vi "Extract Previous Sensor Locations.vi"(8 "error in (no error)":errorcluster, 11 "Folder Path":path) -> (0 "error out":errorcluster, 2 "Smoothness Exam Text":string[][](array[string]), 3 "Sensors":string[][](array[string]))   [LabVIEW 2020]
uses:
  <vilib>/regexp/Match Regular Expression.xnode
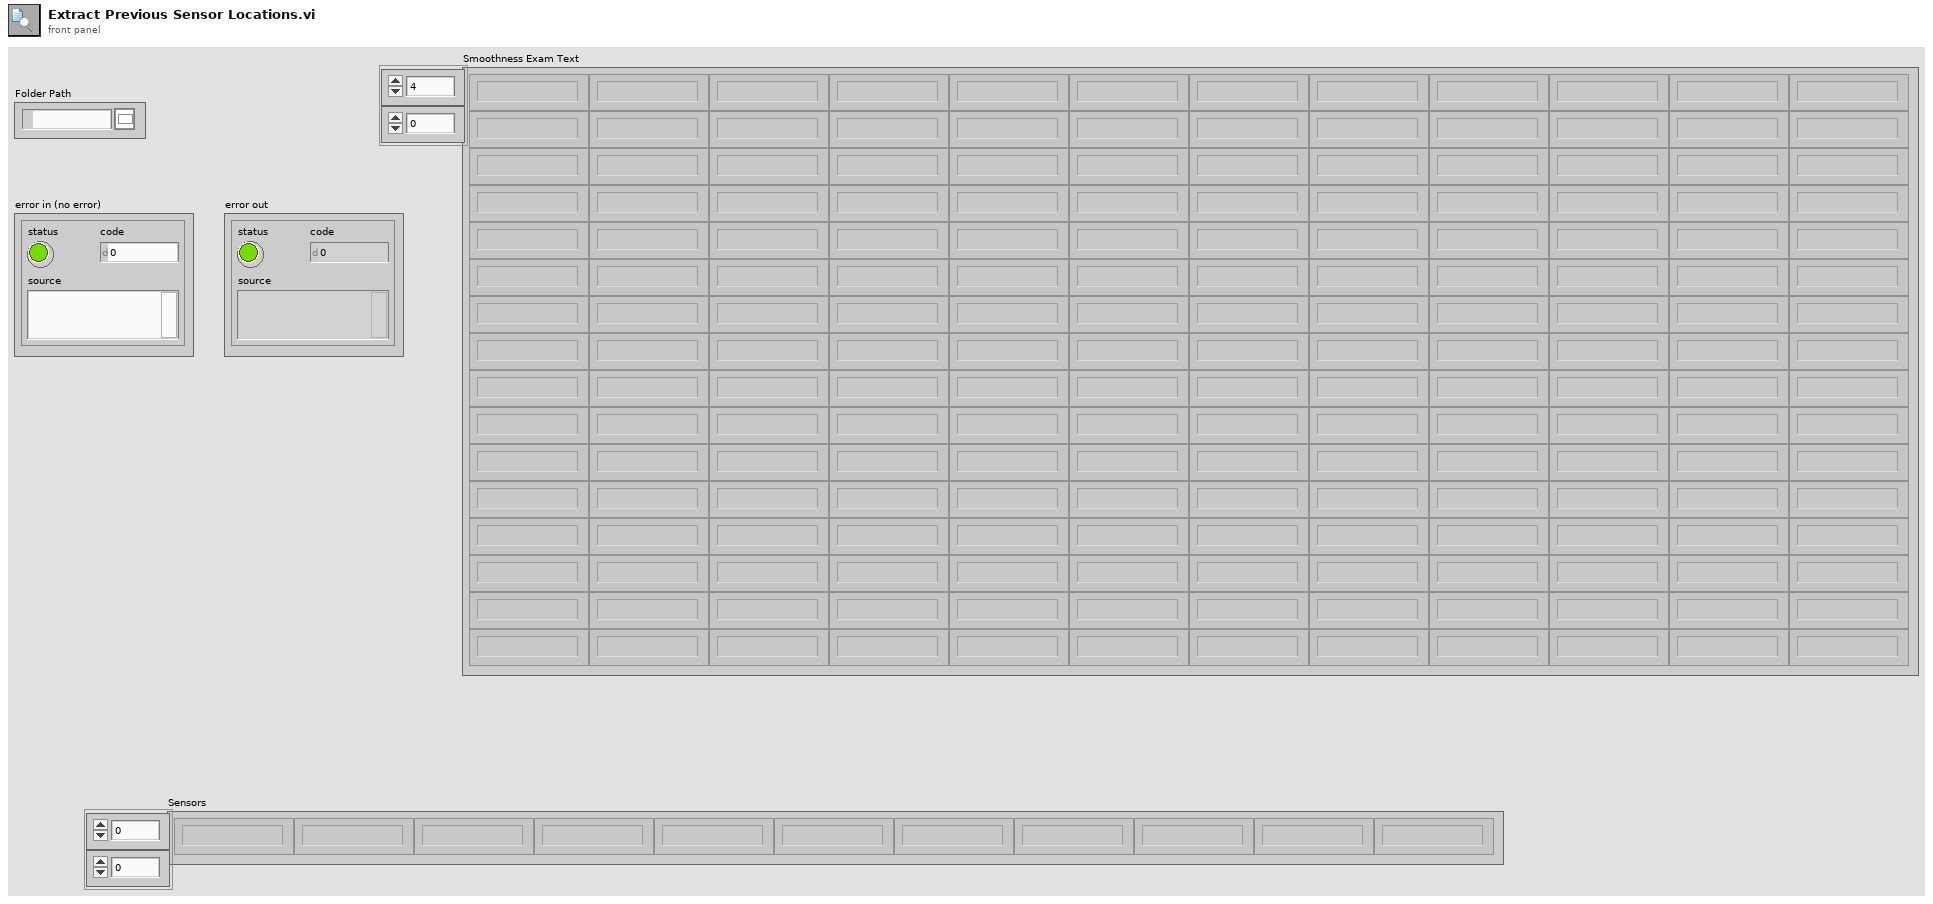
[diagram p1: front panel]
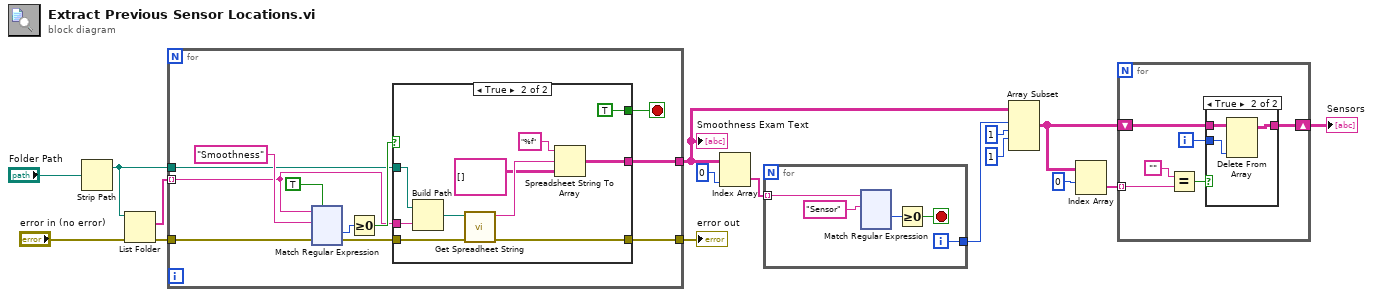
[diagram p0: block diagram]
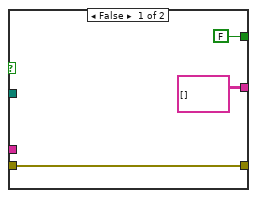
[diagram p3: hidden frame]
diagram:
  n1 = Strip Path(path="Folder Path") -> (stripped path=w12:path)  [unwired: 1 out]
  n2 = List Folder(path=w12, error in="error in (no error)") -> (filenames=w13:string[], error out=w16:errorcluster)  [unwired: 2 in, 2 out]
  n3 = for {
    tunnel: w12 -> [w23]
    tunnel: w13 -> [w22] mode=indexing
    tunnel: [w20] -> w14
    tunnel: w16 -> [w19]
    tunnel: [w18] -> w8
    stop <- w17 stop-if-true
    n4 = xnode "Match Regular Expression"("input string"=w22, "regular expression"="Smoothness", "error in"=w19, "ignore case? (F)"=TRUE) -> ("offset past match"=w24:i32, "error out"=w21:errorcluster)  [unwired: 2 in, 3 out]
    n5 = Greater Or Equal To 0?(x=w24) -> (x >= 0?=w27:bool)
    n6 = case shown="True" w27 {
      tunnel: w22 -> [_ w154]
      tunnel: w23 -> [_ w153]
      tunnel: w21 -> [w144 w151]
      tunnel: [w144 w150] -> w20
      tunnel: [string[][] [] w146] -> w18
      tunnel: [FALSE TRUE] -> w17
      frame False {
      }
      frame True {
        n7 = Build Path(base path=w153, name or relative path=w154) -> (appended path=w152:path)
        n8 = call "Get Spreadheet String.vi"("error in (no error)"=w151, "File Path"=w152) -> ("error out"=w150:errorcluster, "Spreadsheet String"=w148:string)  [unwired: 8 in]
        n9 = Spreadsheet String To Array(format string="%f", spreadsheet string=w148, array type (2D Dbl)=string[][] []) -> (array=w146:string[][])  [unwired: 1 in]
      }
    }
  }
  "error out" <- w14
  "Smoothness Exam Text" <- w8
  n10 = Index Array(array=w8, index (col)=0 ("disabled index (col)")) -> (element=w6:string[])  [unwired: 1 in]
  n11 = for {
    tunnel: w6 -> [w158] mode=indexing
    tunnel: [w159] -> w5
    i -> [w159]
    stop <- w156 stop-if-true
    n12 = xnode "Match Regular Expression"("input string"=w158, "regular expression"="Sensor") -> ("offset past match"=w155:i32)  [unwired: 4 in, 4 out]
    n13 = Greater Or Equal To 0?(x=w155) -> (x >= 0?=w156:bool)
  }
  n14 = Array Subset(array=w8, index (row)=w5, length (row)=1 ("length"), index (col)=1 ("index")) -> (w3:string[][])  [unwired: 1 in]
  n15 = Index Array(array=w3, index (row)=0) -> (element=w2:string[])  [unwired: 1 in]
  n16 = for {
    tunnel: w2 -> [w276] mode=indexing
    shift-right: [w277] -> w4
    shift-left: w3 -> [w279]
    i -> [w278]
    n17 = Equal?(x="", y=w276) -> (x = y?=w275:bool)
    n18 = case shown="True" w275 {
      tunnel: w279 -> [w280 w283]
      tunnel: w278 -> [_ w281]
      tunnel: [w280 w282] -> w277
      frame False {
      }
      frame True {
        n19 = Delete From Array(array=w283, index (col)=w281) -> (array with subset deleted=w282:string[][])  [unwired: 2 in, 1 out]
      }
    }
  }
  "Sensors" <- w4
